vi "全局 2.vi"() -> ()   [LabVIEW 2013]
panel:
  in  "布尔数组 12":bool[](array[boolean])
  in  "布尔数组 11":bool[](array[boolean])
  out "布尔数组 10":bool[](array[boolean])
  out "布尔数组 9":bool[](array[boolean])
  in  "布尔数组 8":bool[](array[boolean])
  in  "布尔数组 7":bool[](array[boolean])
  in  "布尔数组 6":bool[](array[boolean])
  in  "布尔数组 5":bool[](array[boolean])
  out "布尔数组 4":bool[](array[boolean])
  out "布尔数组 3":bool[](array[boolean])
  out "布尔数组 2":bool[](array[boolean])
  out "布尔数组":bool[](array[boolean])
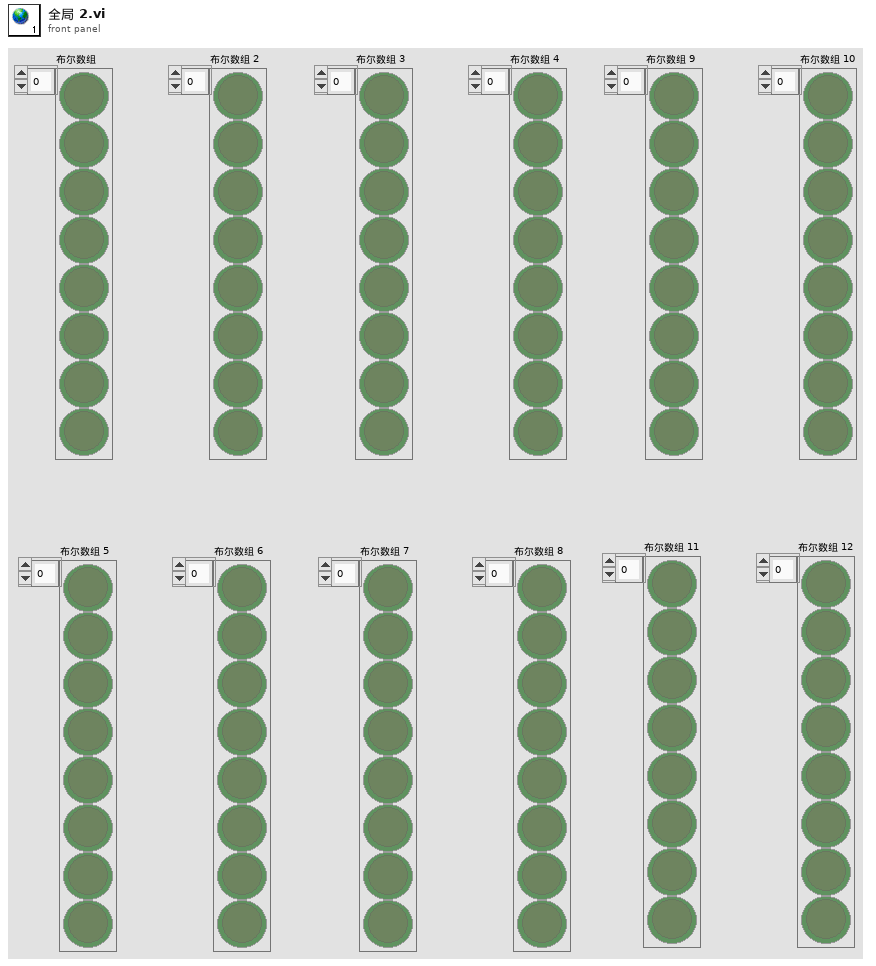
[diagram p1: front panel]
diagram:
